vi "Write Path.vi"(8 "error in":errorcluster, 10 "Path":path=path "approvals", 11 "Namer with Folder in":refnum<class "Namer with Folder.lvclass">) -> (0 "error out":errorcluster, 3 "Namer with Folder out":refnum<class "Namer with Folder.lvclass">)   [LabVIEW 2020, in "Approval Tests.lvlib" / "Namer with Folder.lvclass"]
uses:
  Namer with Folder.lvclass
  Namer with Folder.lvclass/Namer with Folder.ctl
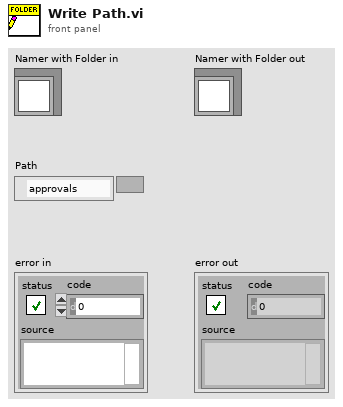
[diagram p1: front panel]
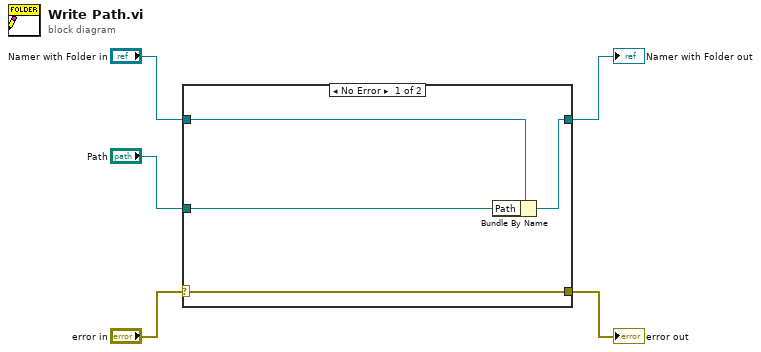
[diagram p0: block diagram]
diagram:
  n1 = case shown="No Error" "error in" {
    selector: "error in" -> [w9 w11]
    tunnel: [w9 w11] -> w4
    tunnel: [w7 w10] -> w2
    tunnel: "Namer with Folder in" -> [w8 w10]
    tunnel: "Path" -> [w6 _]
    frame No Error {
      n2 = Bundle By Name(cluster=w8, "Path"=w6) -> (w7:refnum<class "Namer with Folder.lvclass">)
    }
    frame Error {
    }
  }
  "error out" <- w4
  "Namer with Folder out" <- w2
